vi "Create.vi"(8 "error in (no error)":errorcluster) -> (0 "error out":errorcluster, 3 "GW-PickUp(Half)-Cmd.lvclass":refnum<class "GW-PickUp(Half)-Cmd.lvclass">)   [LabVIEW 2013, in "GW-PickUp(Half)-Cmd.lvclass"]
uses:
  GW-PickUp(Half)-Cmd.lvclass
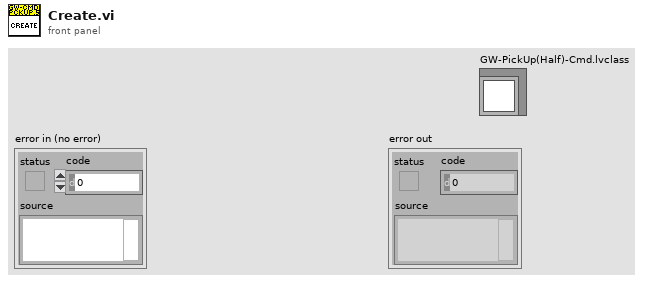
[diagram p1: front panel]
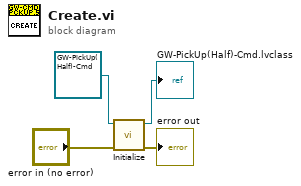
[diagram p0: block diagram]
diagram:
  n1 = call-dynamic "Initialize.vi"("error in (no error)"="error in (no error)", "GW-PickUp(Half)-Cmd in"=refnum<class "GW-PickUp(Half)-Cmd.lvclass"> refnum ("GW-PickUp(Half)-Cmd.lvclass")) -> ("error out"=→"error out":errorcluster, "GW-PickUp(Half)-Cmd out"=→"GW-PickUp(Half)-Cmd.lvclass":refnum<class "GW-PickUp(Half)-Cmd.lvclass">)  [unwired: 8 in]
